vi "Start.vi"(8 "error in (no error)":errorcluster, 11 "selection_dropdown in":refnum<class "selection_dropdown.lvclass">) -> (0 "error out":errorcluster, 3 "selection_dropdown out":refnum<class "selection_dropdown.lvclass">)   [LabVIEW 2024, in "selection_dropdown.lvclass"]
uses:
  selection_dropdown.lvclass
  private/process.vi
  selection_dropdown.lvclass/selection_dropdown.ctl
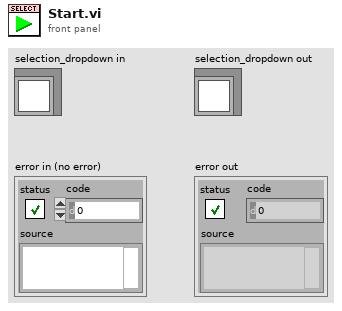
[diagram p1: front panel]
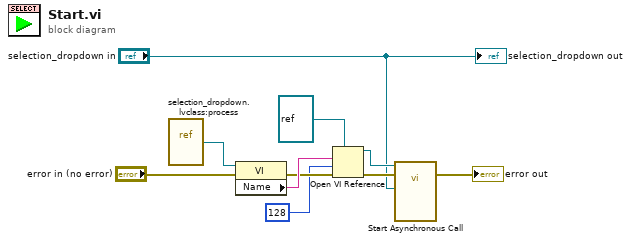
[diagram p0: block diagram]
diagram:
  n1 = vi-ref "selection_dropdown.lvclass:process.vi"() -> (w10:refnum<vi>)
  n2 = property class="VI"(reference=w10, error in="error in (no error)") -> (error out=w8:errorcluster, "Name"=w9:string)  [unwired: 1 out]
  n3 = Open VI Reference(type specifier VI Refnum (for type only)=refnum<vi> refnum, vi path=w9, options=128, error in (no error)=w8) -> (vi reference=w4:refnum<vi>, error out=w5:errorcluster)  [unwired: 2 in]
  n4 = call-by-ref "Start Asynchronous Call"(reference=w4, error in=w5, "class"="selection_dropdown in") -> (error out=→"error out":errorcluster)  [unwired: 11 in, 1 out]
  "selection_dropdown out" <- "selection_dropdown in"
